vi "ASTM Air Data Calculation.vi"(4 "Orifice (mm)":dbl=9.525, 7 "Suction Pressure (kPa)":dbl, 8 "error in (no error)":errorcluster, 9 "Ambient Pressure (kPa) Bt":dbl format="%#_15g", 10 "Ambient Temperature (C)":dbl, 11 "Ambient Humudity (%)":dbl) -> (0 "error out":errorcluster, 2 "Flow-Rate (l/s), Q":dbl, 3 "Suction Power in Air Watt":dbl)   [LabVIEW 2017]
panel:
  out "Flow coefficient K1":dbl
  out "Corrected Suction (kPa), Hs":dbl
  out "Density Ratio, Dr":dbl
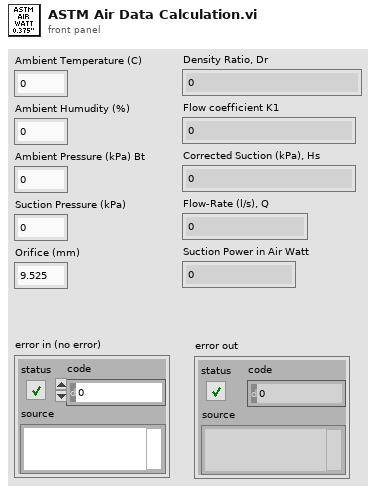
[diagram p1: front panel]
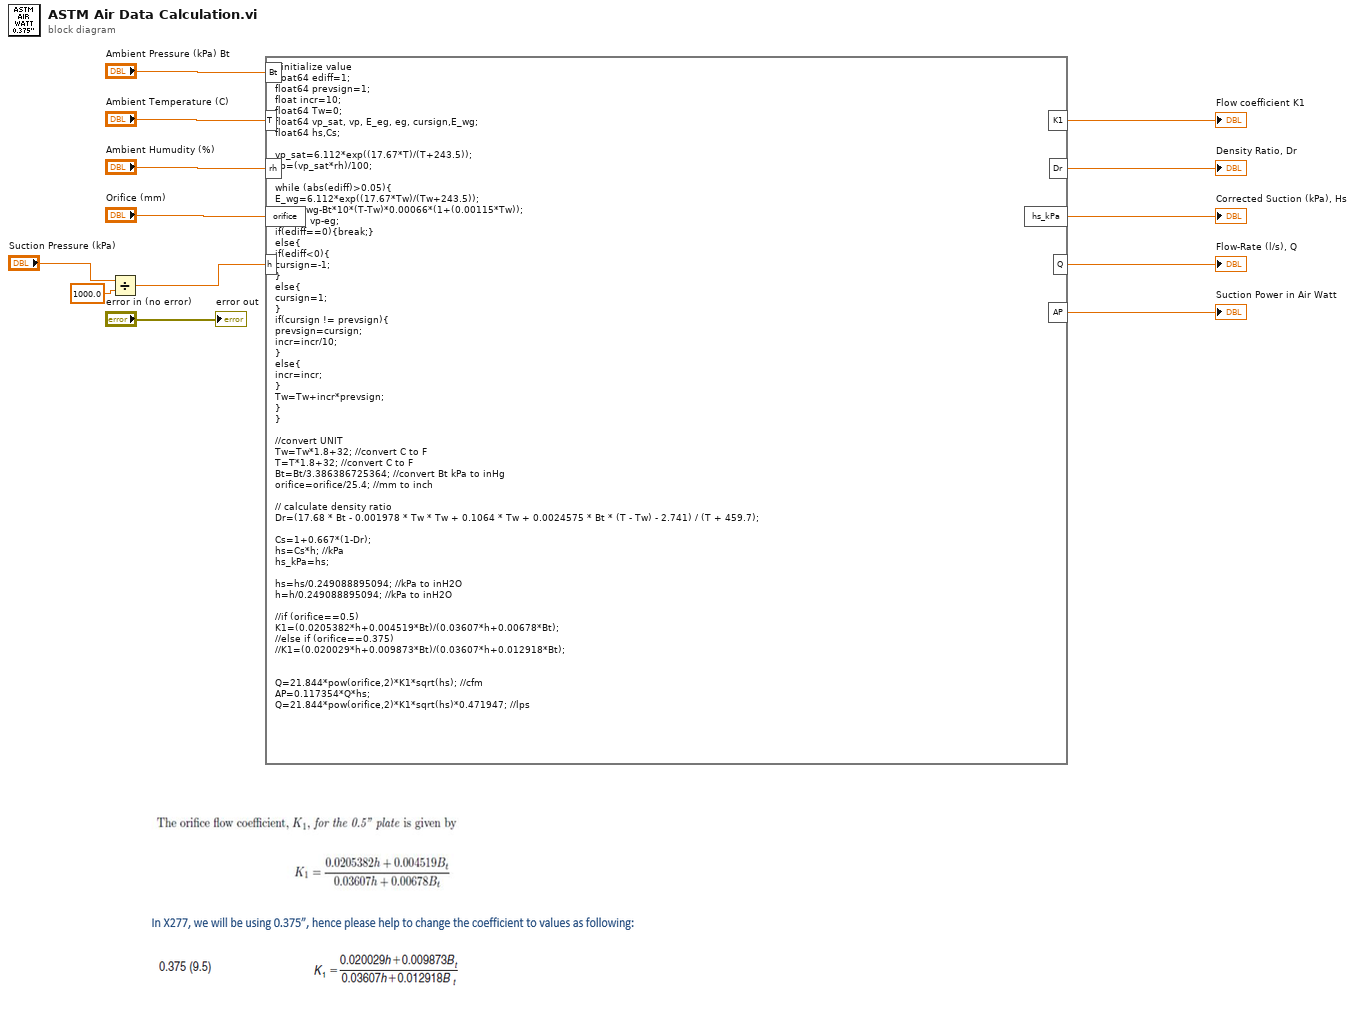
[diagram p0: block diagram]
diagram:
  n1 = Divide(x="Suction Pressure (kPa)", y=1000.0) -> (x/y=w1:dbl)
  n2 = formula code="//initialize value\nfloat64 ediff=1;\nfloat64 prevsign=1;\nfloat incr=10;\nfloat64 Tw=0;\nfloat64 vp_sat, vp, E_eg, eg, cursign,E_wg;\nfloat64 hs,Cs;\n\nvp_sat=6.112*exp((17.67*T)/(T+243.5));\nvp=(vp_sat*rh)/100;\n\nwhile (abs(ediff)>0.05){\nE_wg=6.112*exp((17.67*Tw)/(Tw+243.5));\neg=E_wg-Bt*10*(T-Tw)*0.00066*(1+(0.00115*Tw));\nediff = vp-eg;\nif(ediff==0){break;}\nelse{\nif(ediff<0){\ncursign=-1;\n}\nelse{\ncursign=1;\n}\nif(cursign != prevsign){\nprevsign=cursign;\nincr=incr/10;\n}\nelse{\nincr=incr;\n}\nTw=Tw+incr*prevsign;\n}\n}\n\n//convert UNIT\nTw=Tw*1.8+32; //convert C to F\nT=T*1.8+32; //convert C to F\nBt=Bt/3.386386725364; //convert Bt kPa to inHg\norifice=orifice/25.4; //mm to inch\n\n// calculate density ratio\nDr=(17.68 * Bt - 0.001978 * Tw * Tw + 0.1064 * Tw + 0.0024575 * Bt * (T - Tw) - 2.741) / (T + 459.7);\n\nCs=1+0.667*(1-Dr);\nhs=Cs*h; //kPa\nhs_kPa=hs;\n\nhs=hs/0.249088895094; //kPa to inH2O\nh=h/0.249088895094; //kPa to inH2O\n\n//if (orifice==0.5)\nK1=(0.0205382*h+0.004519*Bt)/(0.03607*h+0.00678*Bt);\n//else if (orifice==0.375)\n//K1=(0.020029*h+0.009873*Bt)/(0.03607*h+0.012918*Bt);\n\n\nQ=21.844*pow(orifice,2)*K1*sqrt(hs); //cfm\nAP=0.117354*Q*hs;\nQ=21.844*pow(orifice,2)*K1*sqrt(hs)*0.471947; //lps"("rh"="Ambient Humudity (%)", "T"="Ambient Temperature (C)", "Bt"="Ambient Pressure (kPa) Bt", "h"=w1, "orifice"="Orifice (mm)") -> ("Dr"=→"Density Ratio, Dr":dbl, "hs_kPa"=→"Corrected Suction (kPa), Hs":dbl, "K1"=→"Flow coefficient K1":dbl, "Q"=→"Flow-Rate (l/s), Q":dbl, "AP"=→"Suction Power in Air Watt":dbl)
  "error out" <- "error in (no error)"
